vi "CalcBouncerGateLEStates.vi"(9 "Bouncer Settings":T1 {"LE12C Voltage" format="%_4f"; "LE13C Voltage" format="%_4f"}, 10 "SampClk.Rate":dbl) -> (1 "Bouncer Waveform":waveform(dbl), 2 "High time":dbl, 3 "low time":dbl)   [LabVIEW 2013]
uses:
  ctl/BouncerParameters.ctl
panel:
  # "ms"
  # "us"
  # "kV"
  # "ms"
  # "us"
  # "kV"
  # "ms"
  # "us"
  # "kV"
  # "ms"
  # "us"
  # "kV"
  # "ms"
  # "us"
  # "kV"
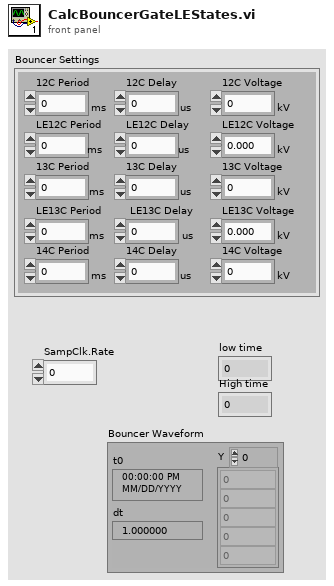
[diagram p1: front panel]
types:
  T1 = typedef "BouncerParameters.ctl" = cluster{"12C Period":dbl, "12C Delay":dbl, "12C Voltage":dbl, "13C Period":dbl, "13C Delay":dbl, "13C Voltage":dbl, "14C Period":dbl, "14C Delay":dbl, "14C Voltage":dbl, "LE13C Period":dbl, "LE13C Delay":dbl, "LE13C Voltage":dbl, "LE12C Period":dbl, "LE12C Delay":dbl, "LE12C Voltage":dbl}
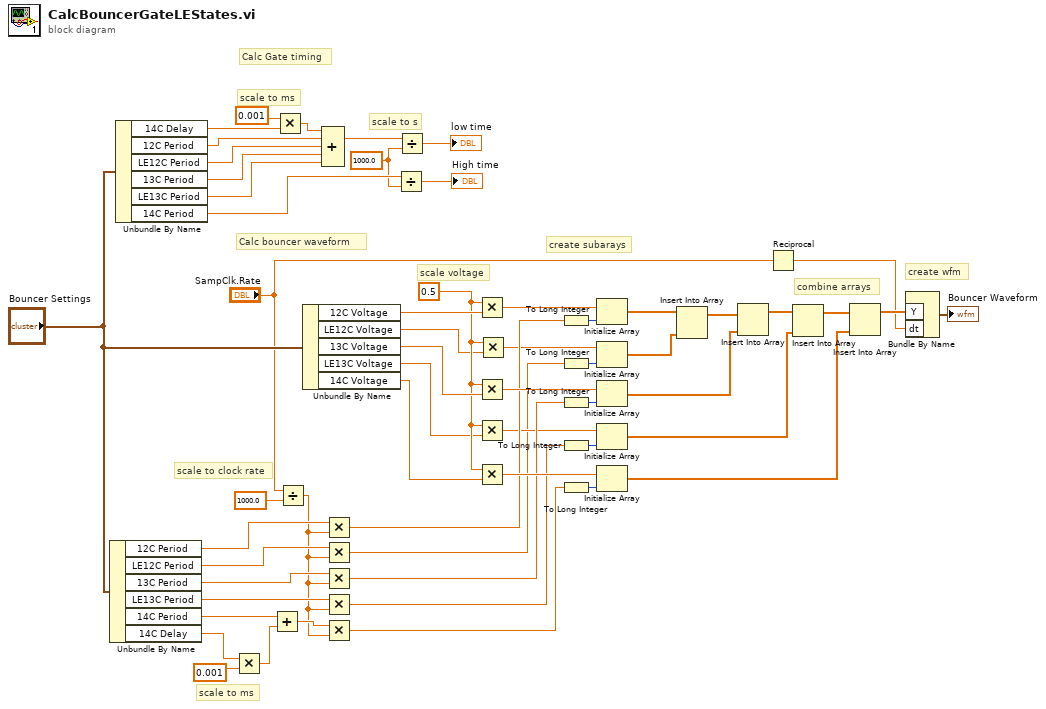
[diagram p0: block diagram]
diagram:
  w32 = 1000.0 ("y")
  w12 = 0.5 ("y")
  # "Calc bouncer waveform"
  # "Calc Gate timing"
  # "create wfm"
  # "combine arrays"
  # "create subarays"
  # "scale voltage"
  # "scale to clock rate"
  # "scale to ms"
  # "scale to s"
  # "scale to ms"
  n1 = Unbundle By Name("Bouncer Settings") -> ("12C Period"=w46:dbl, "LE12C Period"=w5:dbl, "13C Period"=w45:dbl, "LE13C Period"=w4:dbl, "14C Period"=w37:dbl, "14C Delay"=w34:dbl)
  n2 = Unbundle By Name("Bouncer Settings") -> ("14C Delay"=w31:dbl, "12C Period"=w22:dbl, "LE12C Period"=w21:dbl, "13C Period"=w20:dbl, "LE13C Period"=w19:dbl, "14C Period"=w33:dbl)
  n3 = Multiply(x=w34, y=0.001) -> (x*y=w35:dbl)
  n4 = Add(x=w37, y=w35) -> (x+y=w57:dbl)
  n5 = Multiply(x=0.001 ("y"), y=w31) -> (x*y=w23:dbl)
  n6 = Divide(x="SampClk.Rate", y=1000.0) -> (x/y=w3:dbl)
  n7 = Unbundle By Name("Bouncer Settings") -> ("12C Voltage"=w44:dbl, "LE12C Voltage"=w11:dbl, "13C Voltage"=w43:dbl, "LE13C Voltage"=w9:dbl, "14C Voltage"=w42:dbl)
  n8 = Compound Arithmetic op=ADD(w23, w22, w21, w20, w19) -> (w24:dbl)
  n9 = Multiply(x=w46, y=w3) -> (x*y=w50:dbl)
  n10 = Multiply(x=w5, y=w3) -> (x*y=w1:dbl)
  n11 = Multiply(x=w45, y=w3) -> (x*y=w49:dbl)
  n12 = Multiply(x=w4, y=w3) -> (x*y=w2:dbl)
  n13 = Multiply(x=w57, y=w3) -> (x*y=w48:dbl)
  n14 = Divide(x=w33, y=w32) -> (x/y=→"High time":dbl)
  n15 = Divide(x=w24, y=w32) -> (x/y=→"low time":dbl)
  n16 = Multiply(x=w12, y=w44) -> (x*y=w55:dbl)
  n17 = Multiply(x=w12, y=w43) -> (x*y=w54:dbl)
  n18 = Multiply(x=w12, y=w9) -> (x*y=w8:dbl)
  n19 = Multiply(x=w12, y=w42) -> (x*y=w56:dbl)
  n20 = Multiply(x=w12, y=w11) -> (x*y=w10:dbl)
  n21 = To Long Integer(number=w50) -> (32bit integer=w39:i32)
  n22 = To Long Integer(number=w1) -> (32bit integer=w18:i32)
  n23 = To Long Integer(number=w49) -> (32bit integer=w40:i32)
  n24 = To Long Integer(number=w2) -> (32bit integer=w17:i32)
  n25 = To Long Integer(number=w48) -> (32bit integer=w41:i32)
  n26 = Initialize Array(w55, w39) -> (w16:dbl[])
  n27 = Initialize Array(w10, w18) -> (w7:dbl[])
  n28 = Initialize Array(w54, w40) -> (w53:dbl[])
  n29 = Initialize Array(w8, w17) -> (w6:dbl[])
  n30 = Initialize Array(w56, w41) -> (w52:dbl[])
  n31 = Insert Into Array(array=w16, new element=w7) -> (w15:dbl[])  [unwired: 1 in]
  n32 = Insert Into Array(array=w15, new element=w53) -> (w14:dbl[])  [unwired: 1 in]
  n33 = Reciprocal(x="SampClk.Rate") -> (1/x=w47:dbl)
  n34 = Insert Into Array(array=w14, new element=w6) -> (w13:dbl[])  [unwired: 1 in]
  n35 = Insert Into Array(array=w13, new element=w52) -> (w51:dbl[])  [unwired: 1 in]
  n36 = Bundle By Name("Y"=w51, "dt"=w47) -> (→"Bouncer Waveform":waveform(dbl))  [unwired: 1 out]
